vi "chopper MC2000B.vi"() -> ()   [LabVIEW 2024]
uses:
  <instrlib>/Thorlabs_MC2000B/Thorlabs_MC2000B.lvlib
panel:
  in  "Frequency (Hz)":i32
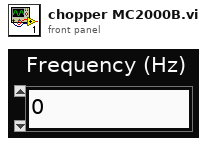
[diagram p1: front panel]
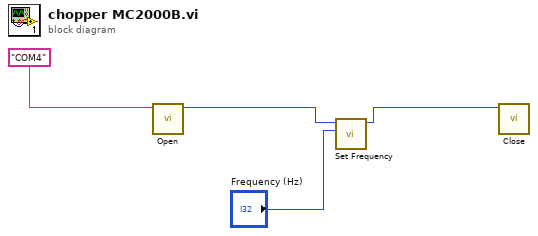
[diagram p0: block diagram]
diagram:
  n1 = call <instrlib>:"Open.vi"("Serial Port"="COM4") -> ("Handle out"=w1:i32)  [unwired: 8 in, 2 out]
  n2 = call <instrlib>:"Set Frequency.vi"("Frequency (Hz)"="Frequency (Hz)", "Handle in"=w1) -> ("Handle out"=w3:i32)  [unwired: 8 in, 1 out]
  n3 = call <instrlib>:"Close.vi"("hdl"=w3) -> ()  [unwired: 10 in, 1 out]
